vi "check manifold config array value errors (sub-vi).vi"(7 "odor config array":T8, 10 "manifold config array":T1) -> (2 "manifold config error flag array":bool[][](array[boolean]), 4 "value error out":errorcluster)   [LabVIEW 2021]
uses:
  type-defs/odor description array (type def).ctl
  type-defs/odor info cluster (type def).ctl
  type-defs/odor selection (type def).ctl
  type-defs/odor color (type def).ctl
  type-defs/manifold configuration cluster array (type def).ctl
  type-defs/manifold configuration cluster (type def).ctl
  type-defs/manifold selection.ctl
  type-defs/single port single odor cluster.ctl
  type-defs/port number (type def).ctl
  <vilib>/ErrorRing/Error Ring.xnode
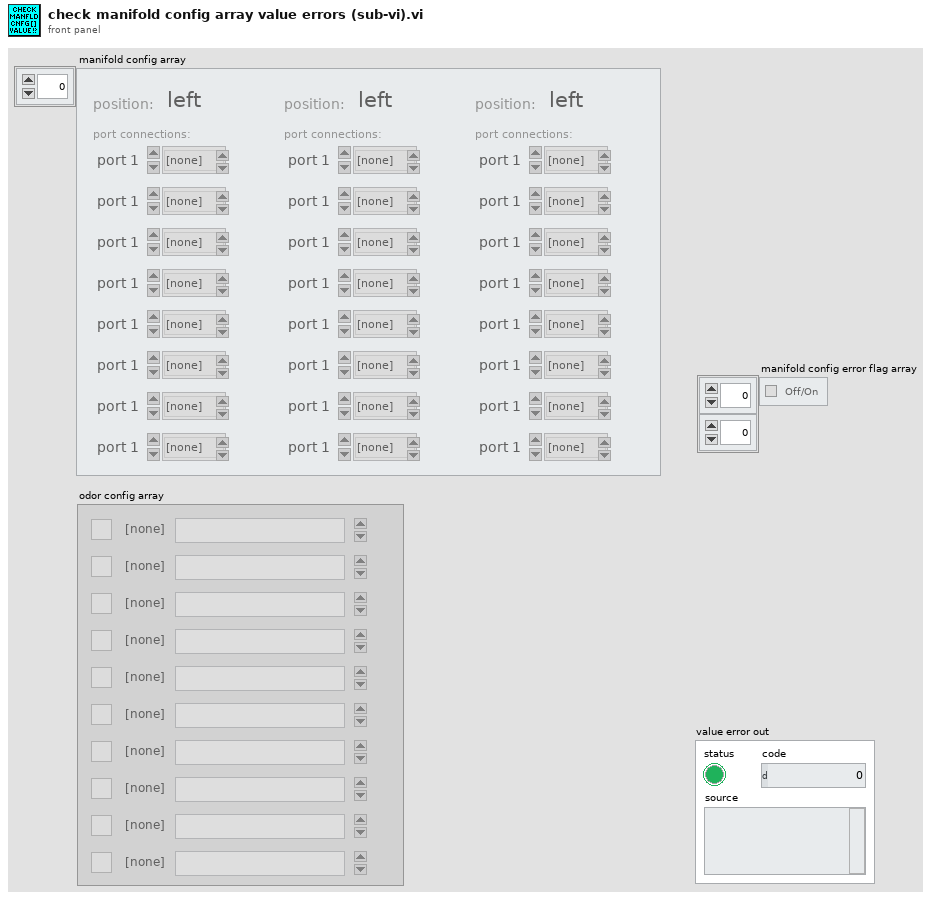
[diagram p1: front panel]
types:
  T1 = typedef "manifold configuration cluster array (type def).ctl" = T2[]
  T2 = typedef "manifold configuration cluster (type def).ctl" = cluster{"position:":T3, "port connections:":T4[]}
  T3 = typedef "manifold selection.ctl" = enum16{"left", "middle", "right"}
  T4 = typedef "single port single odor cluster.ctl" = cluster{"port number":T5, "connected odor":T6, "error":bool, "odor color":T7}
  T5 = typedef "port number (type def).ctl" = enum16{"port 1", "port 2", "port 3", "port 4", "port 5", "port 6", "port 7", "port 8"}
  T6 = typedef "odor selection (type def).ctl" = enum16{"[none]", "odor 1", "odor 2", "odor 3", "odor 4", "odor 5", "odor 6", "odor 7", "odor 8", "odor 9", "odor 10"}
  T7 = typedef "odor color (type def).ctl" = u16
  T8 = typedef "odor description array (type def).ctl" = T9[]
  T9 = typedef "odor info cluster (type def).ctl" = cluster{"odor channel":T6, "odor description":string, "odor color":T7, "odor channel active":bool}
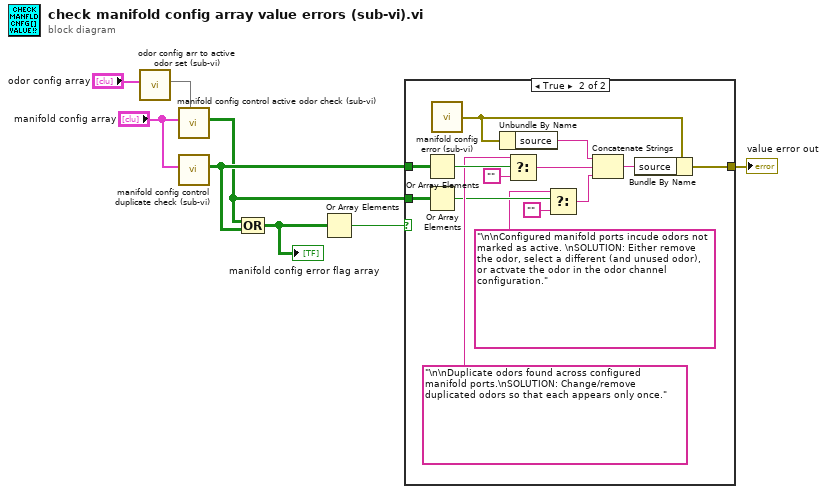
[diagram p0: block diagram]
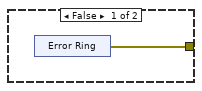
[diagram p2: hidden frame]
diagram:
  n1 = call "odor config arr to active odor set (sub-vi).vi"("odor descriptions"="odor config array") -> ("active odor chanel set"=w2:set{T6})  [unwired: 10 in]
  n2 = call "manifold config control active odor check (sub-vi).vi"("active odor chanel set"=w2, "manifold config array"="manifold config array") -> ("manifold config error flag array"=w3:bool[][])  [unwired: 9 in]
  n3 = call "manifold config control duplicate check (sub-vi).vi"("manifold config array"="manifold config array") -> ("manifold config error flag array"=w4:bool[][])  [unwired: 10 in]
  n4 = Compound Arithmetic op=OR(w3, w4) -> (w7:bool[][])
  "manifold config error flag array" <- w7
  n5 = Or Array Elements(Boolean array=w7) -> (logical OR=w6:bool)
  n6 = case shown="True" w6 {
    tunnel: [w9 w11] -> w5
    tunnel: w4 -> [_ w24]
    tunnel: w3 -> [_ w23]
    frame False {
      n7 = xnode "Error Ring"() -> ("error out"=w9:errorcluster)
    }
    frame True {
      n8 = Or Array Elements(Boolean array=w24) -> (logical OR=w22:bool)
      n9 = Or Array Elements(Boolean array=w23) -> (logical OR=w16:bool)
      n10 = call "manifold config error (sub-vi).vi"() -> ("error"=w13:errorcluster)  [unwired: 1 in]
      n11 = Unbundle By Name(w13) -> ("source"=w20:string)
      n12 = Select(t="\n\nDuplicate odors found across configured manifold ports.\nSOLUTION: Change/remove duplicated odors so that each appears only once.", s=w22, f="") -> (s? t:f=w19:string)
      n13 = Select(t="\n\nConfigured manifold ports incude odors not marked as active. \nSOLUTION: Either remove the odor, select a different (and unused odor), or actvate the odor in the odor channel configuration.", s=w16, f="") -> (s? t:f=w14:string)
      n14 = Concatenate Strings(w20, w19, w14) -> (w12:string)
      n15 = Bundle By Name(cluster=w13, "source"=w12) -> (w11:errorcluster)
    }
  }
  "value error out" <- w5
